vi "zapisNowy.vi"(0 "Byte Stream File Refnum in":refnum<file>, 1 "thin":dbl, 3 "thout":dbl, 7 "Typ in":string, 11 "error in (no error)":errorcluster, 12 "Zapis do pliku":bool, 13 "probka in":dbl) -> (4 "Byte Stream File Refnum out":refnum<file>, 15 "error out":errorcluster)   [LabVIEW 2023]
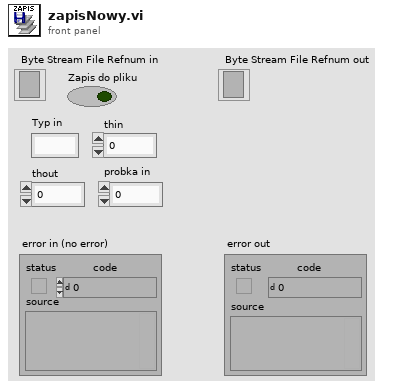
[diagram p1: front panel]
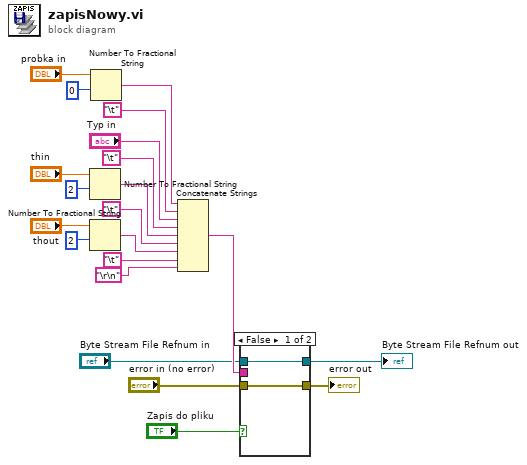
[diagram p0: block diagram]
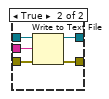
[diagram p2: hidden frame]
diagram:
  n1 = Number To Fractional String(number="thin", precision (6)=i16 2) -> (F-format string=w5:string)  [unwired: 2 in]
  n2 = Number To Fractional String(number="thout", precision (6)=i16 2) -> (F-format string=w3:string)  [unwired: 2 in]
  n3 = Number To Fractional String(number="probka in", precision (6)=i16 0) -> (F-format string=w9:string)  [unwired: 2 in]
  n4 = Concatenate Strings(w9, "\t", "Typ in", "\t", w5, "\t", w3, "\t", "\r\n") -> (w21:string)
  n5 = case shown="False" "Zapis do pliku" {
    tunnel: w21 -> [_ w28]
    tunnel: "Byte Stream File Refnum in" -> [w22 w27]
    tunnel: "error in (no error)" -> [w23 w26]
    tunnel: [w23 w25] -> w17
    tunnel: [w22 w24] -> w16
    frame False {
    }
    frame True {
      n6 = Write to Text File(file (use dialog)=w27, text=w28, error in=w26) -> (refnum out=w24:refnum<file>, error out=w25:errorcluster)  [unwired: 1 in, 1 out]
    }
  }
  "error out" <- w17
  "Byte Stream File Refnum out" <- w16
